vi "SQLiteLCOD.vi"(4 "dB Command":T2, 5 "error in (no error)":errorcluster, 7 "Waveform":T1, 8 "String":string) -> (0 "error out":errorcluster, 3 "Rows":string[][](array[string]))   [LabVIEW 2023, in "SQLiteLCOD.lvlib"]
doc: "For Change Password use $$ string as below\nFilepath to db3 file$$oldpassword$$newpassword\n\neg\n\nC:\\Users\\Public\\SSDC\\GenApp2013-b\\Project\\SourceCode\\Config.db3$$$$guessme\n\nwill set up a password of \"guessme\" on an unprotected db3 file \n\nTo open a password protected db us the following\nC:\\Users\\Public\\SSDC\\GenApp2013-b\\Project\\SourceCode\\Config.db3->guessme"
uses:
  SQLiteLCOD.lvlib
  SQLITE/SQL Connection/Connection.lvclass
  SQLITE/SQL Connection/Open (string).vi
  SQLITE/SQL Statement/SQL Statement.lvclass
  SQLiteLCOD.ctl
  Waveform.ctl
panel:
  # "Input"
  # "Output"
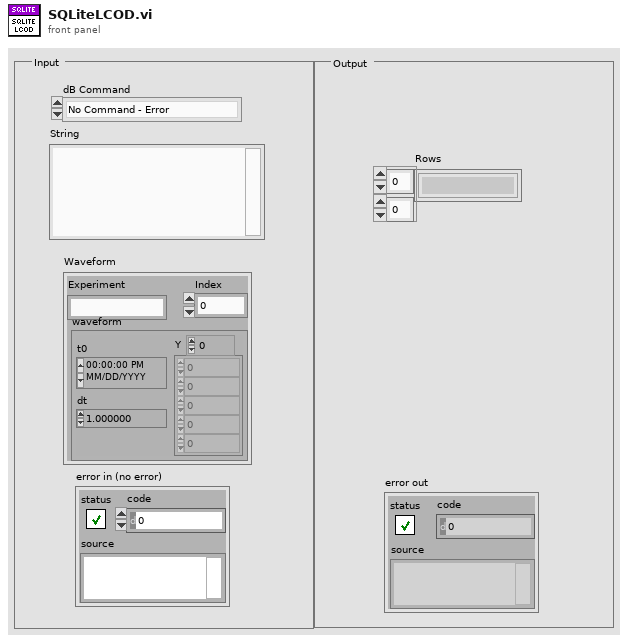
[diagram p1: front panel]
types:
  T1 = typedef "Waveform.ctl" = cluster{"Experiment":string, "Index":u32, "waveform":waveform(dbl)}
  T2 = typedef "SQLiteLCOD.lvlib/SQLiteLCOD.ctl" = enum16{"No Command - Error", "Open", "SQL", "Close", "Prepare SQL", "INSERT Waveform", "INSERT LongText", "Finalise SQL"}
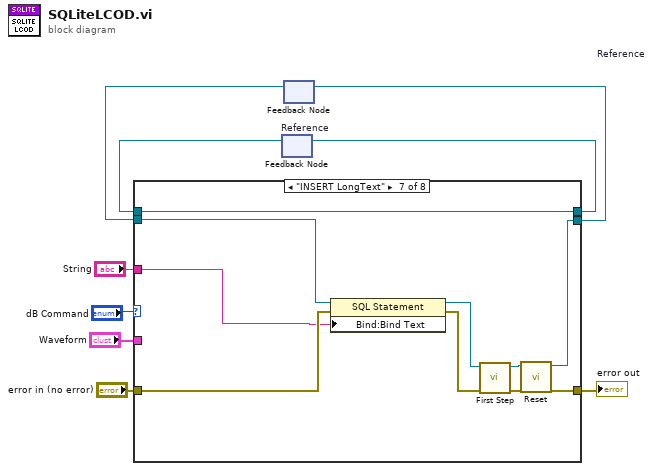
[diagram p0: block diagram]
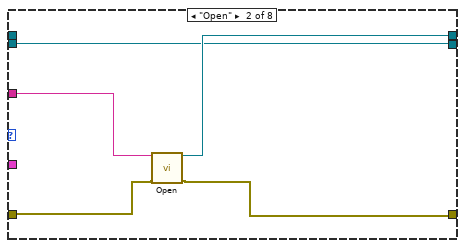
[diagram p3: hidden frame]
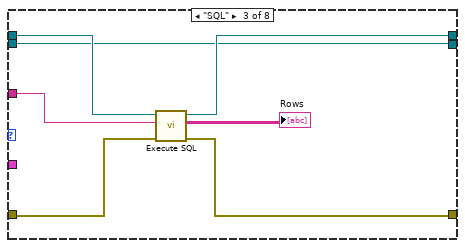
[diagram p4: hidden frame]
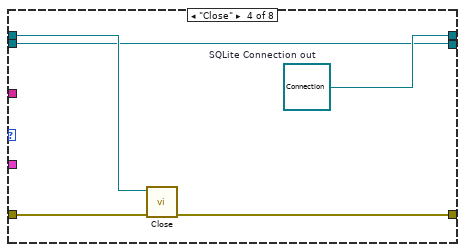
[diagram p5: hidden frame]
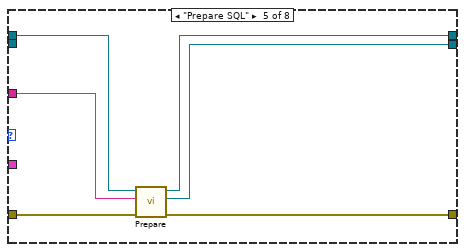
[diagram p6: hidden frame]
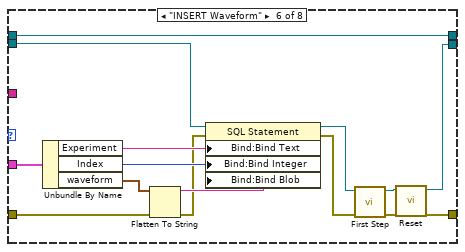
[diagram p7: hidden frame]
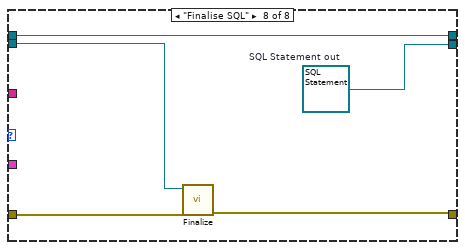
[diagram p8: hidden frame]
diagram:
  n1 = feedback #1 "Reference"() -> (w4:refnum<class "Connection.lvclass">)  [unwired: 1 in]
  n2 = feedback #2 "Reference"() -> (w2:refnum<class "SQL Statement.lvclass">)  [unwired: 1 in]
  n3 = case shown="\"INSERT LongText\"" "dB Command" {
    tunnel: "error in (no error)" -> [w12 w16 w20 w27 w34 w42 w52 w64]
    tunnel: "String" -> [_ w14 w23 _ w33 _ w51 _]
    tunnel: [w12 w17 w21 w28 w30 w41 w58 w62] -> w6
    tunnel: [w11 w15 w19 w29 w32 w50 w60 w65] -> w5
    tunnel: w4 -> [w11 _ w24 w26 w35 w50 w60 w65]
    tunnel: [w10 w13 w18 w25 w31 w38 w55 w61] -> w3
    tunnel: w2 -> [w10 w13 w18 w25 _ w49 w59 w63]
    tunnel: "Waveform" -> [_ _ _ _ _ w48 _ _]
    frame "No Command - Error", Default {
    }
    frame "Open" {
      n4 = call-poly "Open.vi"("error in (no error)"=w16, "db file"=w14) -> ("error out"=w17:errorcluster, "SQLite Connection out"=w15:refnum<class "Connection.lvclass">)  [unwired: 8 in]
    }
    frame "SQL" {
      n5 = call "Execute SQL.vi"("error in (no error)"=w20, "SQL"=w23, "SQLite Connection in"=w24) -> ("error out"=w21:errorcluster, "Result Set"=→"Rows":string[][], "SQLite Connection out"=w19:refnum<class "Connection.lvclass">)  [unwired: 5 in, 1 out]
    }
    frame "Close" {
      w29 = refnum<class "Connection.lvclass"> refnum  # SQLite Connection out
      n6 = call "Close.vi"("error in (no error)"=w27, "SQLite Connection in"=w26) -> ("error out"=w28:errorcluster)  [unwired: 9 in]
    }
    frame "Prepare SQL" {
      n7 = call "Prepare.vi"("error in (no error)"=w34, "SQL"=w33, "SQLite Connection in"=w35) -> ("error out"=w30:errorcluster, "SQL Statement out"=w31:refnum<class "SQL Statement.lvclass">, "SQLite Connection out"=w32:refnum<class "Connection.lvclass">)  [unwired: 4 in, 2 out]
    }
    frame "INSERT Waveform" {
      n8 = Unbundle By Name(w48) -> ("Experiment"=w47:string, "Index"=w46:u32, "waveform"=w45:waveform(dbl))
      n9 = Flatten To String(anything=w45, error in (no error)=w42) -> (data string=w44:string, error out=w43:errorcluster)  [unwired: 2 in, 1 out]
      n10 = property class="SQL Statement"(reference=w49, error in=w43, "Bind:Bind Text"=w47, "Bind:Bind Integer"=w46, "Bind:Bind Blob"=w44) -> (reference out=w37:refnum<class "SQL Statement.lvclass">, error out=w40:errorcluster)
      n11 = call "First Step.vi"("error in (no error)"=w40, "SQL Statement in"=w37) -> ("error out"=w39:errorcluster, "SQL Statement out"=w36:refnum<class "SQL Statement.lvclass">)  [unwired: 7 in, 1 out]
      n12 = call "Reset.vi"("error in (no error)"=w39, "SQL Statement in"=w36) -> ("error out"=w41:errorcluster, "SQL Statement out"=w38:refnum<class "SQL Statement.lvclass">)  [unwired: 8 in]
    }
    frame "INSERT LongText" {
      n13 = property class="SQL Statement"(reference=w59, error in=w52, "Bind:Bind Text"=w51) -> (reference out=w54:refnum<class "SQL Statement.lvclass">, error out=w57:errorcluster)
      n14 = call "First Step.vi"("error in (no error)"=w57, "SQL Statement in"=w54) -> ("error out"=w56:errorcluster, "SQL Statement out"=w53:refnum<class "SQL Statement.lvclass">)  [unwired: 7 in, 1 out]
      n15 = call "Reset.vi"("error in (no error)"=w56, "SQL Statement in"=w53) -> ("error out"=w58:errorcluster, "SQL Statement out"=w55:refnum<class "SQL Statement.lvclass">)  [unwired: 8 in]
    }
    frame "Finalise SQL" {
      w61 = refnum<class "SQL Statement.lvclass"> refnum  # SQL Statement out
      n16 = call "Finalize.vi"("error in (no error)"=w64, "SQL Statement in"=w63) -> ("error out"=w62:errorcluster)  [unwired: 9 in]
    }
  }
  "error out" <- w6
  n17 = feedback-in #1(w5) -> ()
  n18 = feedback-in #2(w3) -> ()
